vi "5_2.vi"() -> ()   [LabVIEW 2017]
panel:
  out "Time [ms]":u32
  out "Waveform Chart":dbl(graph)
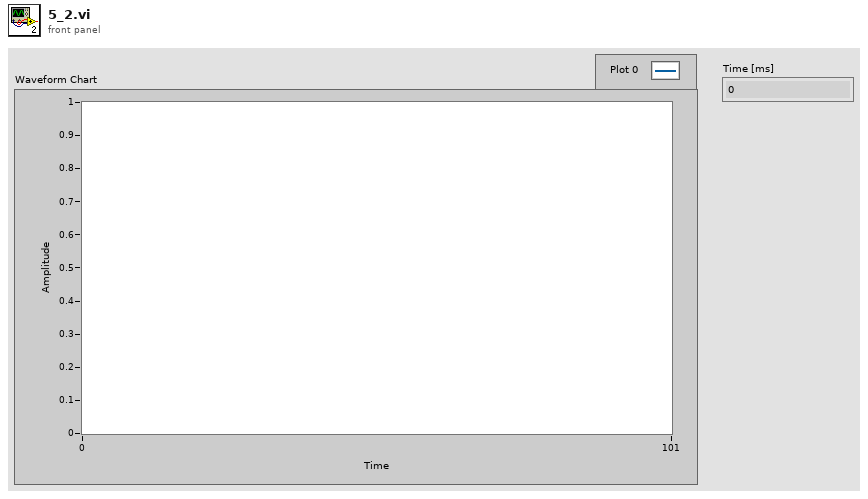
[diagram p1: front panel]
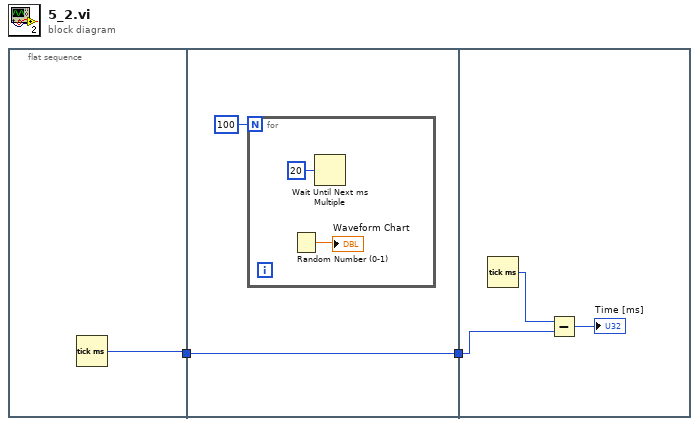
[diagram p0: block diagram]
diagram:
  n1 = flat-sequence {
    tunnel: [w3] -> w2
    tunnel: w2 -> [w4]
    tunnel: [w4] -> w1
    tunnel: w1 -> [w10]
    frame #0 {
      n2 = Tick Count (ms)() -> (millisecond timer value=w3:u32)
    }
    frame #1 {
      n3 = for {
        N: 100 -> [_]
        n4 = Random Number (0-1)() -> (number: 0 to 1=→"Waveform Chart":dbl)
        n5 = Wait Until Next ms Multiple(millisecond multiple=u32 20) -> ()  [unwired: 1 out]
      }
    }
    frame #2 {
      n6 = Tick Count (ms)() -> (millisecond timer value=w9:u32)
      n7 = Subtract(x=w9, y=w10) -> (x-y=→"Time [ms]":u32)
    }
  }
